vi "File.Log File Content Error Check.vi"(6 "Error Msg Prefix":string[](array[string])=["ERROR:"], 8 "error in (no error)":errorcluster, 9 "Fault Code":i32=-4000, 10 "Test Name":string, 11 "Log File Path":path) -> (0 "error out":errorcluster)   [LabVIEW 2024]
uses:
  Errors/Error.Error Code List.ctl
  <vilib>/Utility/error.llb/Trim Whitespace One-Sided.vi
  <vilib>/KATE/Files/File Utils.lvlib
  Errors.lvlib
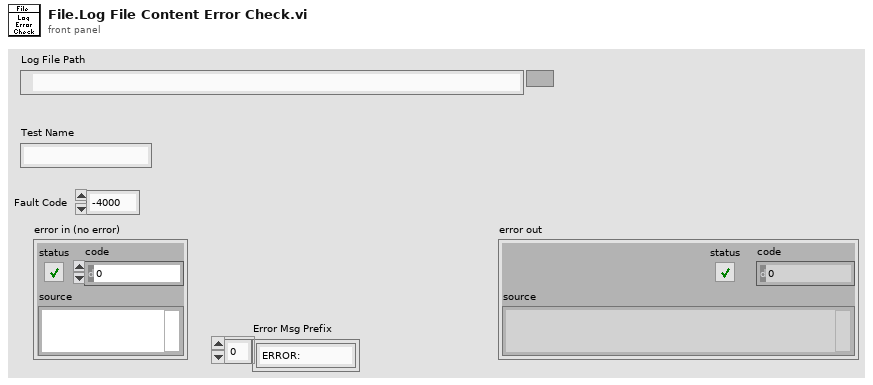
[diagram p1: front panel]
types:
  T1 = typedef "EQMF.lvlib/Errors.lvlib/Error.Error Code List.ctl" = i32
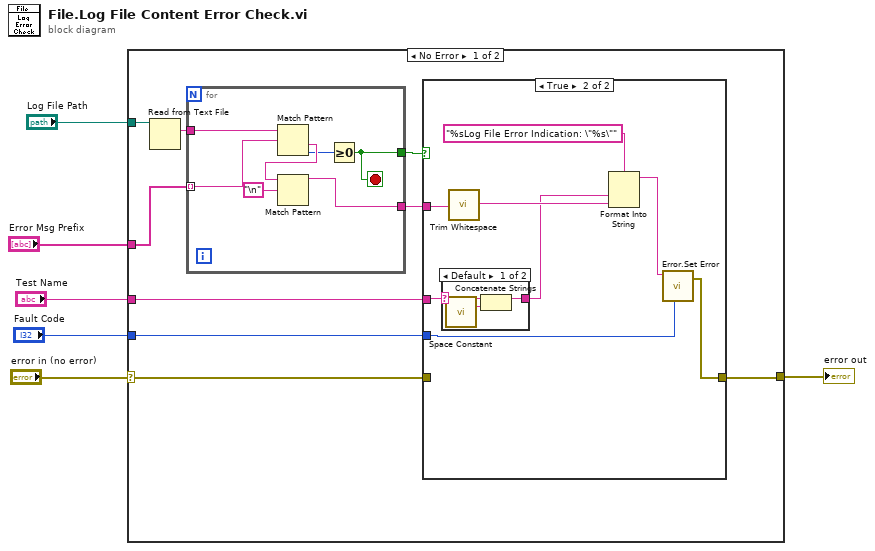
[diagram p0: block diagram]
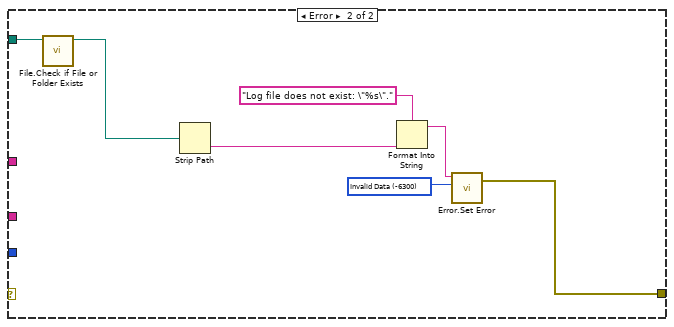
[diagram p4: hidden frame]
diagram:
  n1 = case shown="No Error" "error in (no error)" {
    selector: "error in (no error)" -> [w10 _]
    tunnel: "Log File Path" -> [w15 w41]
    tunnel: [w9 w35] -> w5
    tunnel: "Error Msg Prefix" -> [w12 _]
    tunnel: "Fault Code" -> [w8 _]
    tunnel: "Test Name" -> [w7 _]
    frame No Error {
      n2 = Read from Text File(file (use dialog)=w15) -> (text=w14:string)  [unwired: 3 in, 3 out]
      n3 = for {
        tunnel: w14 -> [w22]
        tunnel: [w18] -> w13
        tunnel: w12 -> [w17] mode=indexing
        tunnel: [w16] -> w11
        stop <- w18 stop-if-true
        n4 = Match Pattern(string=w22, regular expression=w17) -> (after substring=w21:string, offset past match=w19:i32)  [unwired: 1 in, 2 out]
        n5 = Match Pattern(string=w21, regular expression="\n") -> (before substring=w16:string)  [unwired: 1 in, 3 out]
        n6 = Greater Or Equal To 0?(x=w19) -> (x >= 0?=w18:bool)
      }
      n7 = case shown="True" w13 {
        tunnel: w11 -> [_ w30]
        tunnel: w10 -> [_ _]
        tunnel: [_ w23] -> w9
        tunnel: w8 -> [_ w24]
        tunnel: w7 -> [_ w26]
        frame False {
        }
        frame True {
          n8 = case shown="Default" w26 {
            selector: w26 -> [w33 w34]
            tunnel: [w32 w34] -> w25
            frame Default {
              n9 = call <vilib>:"Space Constant.vi"() -> ("String"=w31:string)
              n10 = Concatenate Strings(w33, w31) -> (w32:string)
            }
            frame "" {
            }
          }
          n11 = call <vilib>:"Trim Whitespace.vi"("string"=w30) -> ("trimmed string"=w27:string)  [unwired: 1 in]
          n12 = Format Into String(format string="%sLog File Error Indication: \"%s\"", w25, w27) -> (resulting string=w28:string)  [unwired: 2 in, 1 out]
          n13 = call "Error.Set Error.vi"("Code"=w24, "Desc"=w28) -> ("error out"=w23:errorcluster)  [unwired: 5 in]
        }
      }
    }
    frame Error {
      w36 = T1 -6300 items=["No Error"=0, "Abort"=-2, "Misc"=-5000, "Fixture Error"=-5100, "File IO - General"=-5200, "FIle IO - Config Error"=-5201, "Instrument - General"=-5300, "Instrument - Serial Com"=-5301, "Instrument - Camera"=-5302, "Instrument - PS"=-5303, "Instrument - Oscilloscope"=-5304, "Instrument - Function Gen"=-5305, "Instrument - Load"=-5306, "Instrument - Meter"=-5307, "Instrument - Power Control"=-5308, "Instrument - Motion"=-5309, "Instrument - RF"=-5310, "System Exe"=-5400, "Image Processing"=-5500, "Communication"=-5600, "Script - Syntax Error"=-6000, "Script - Invalid Name or Param"=-6100, "Script - Timeout"=-6200, "Invalid Data"=-6300, "FW Update Error"=-6500] ("Std Code")
      n14 = call <vilib>:"File.Check if File or Folder Exists.vi"("Path"=w41) -> ("Dup Path"=w40:path)  [unwired: 6 in, 4 out]
      n15 = Strip Path(path=w40) -> (name=w38:string)  [unwired: 1 out]
      n16 = Format Into String(format string="Log file does not exist: \"%s\".", w38) -> (resulting string=w37:string)  [unwired: 2 in, 1 out]
      n17 = call "Error.Set Error.vi"("Std Code"=w36, "Desc"=w37) -> ("error out"=w35:errorcluster)  [unwired: 5 in]
    }
  }
  "error out" <- w5
